vi "Read Roles.vi"(8 "error in (no error)":errorcluster, 11 "KickPenaltyAllyPlay in":refnum<class "KickPenaltyAllyPlay.lvclass">) -> (0 "error out":errorcluster, 2 "Roles":T1, 3 "KickPenaltyAllyPlay out":refnum<class "KickPenaltyAllyPlay.lvclass">)   [LabVIEW 2023, in "KickPenaltyAllyPlay.lvclass"]
uses:
  KickPenaltyAllyPlay.lvclass
  kickPenaltyAllyRoles.ctl
  PenaltyAttackerRole_class/PenaltyAttackerRole.lvclass
  HaltRole_class/HaltRole.lvclass
  KickPenaltyAllyPlay.lvclass/KickPenaltyAllyPlay.ctl
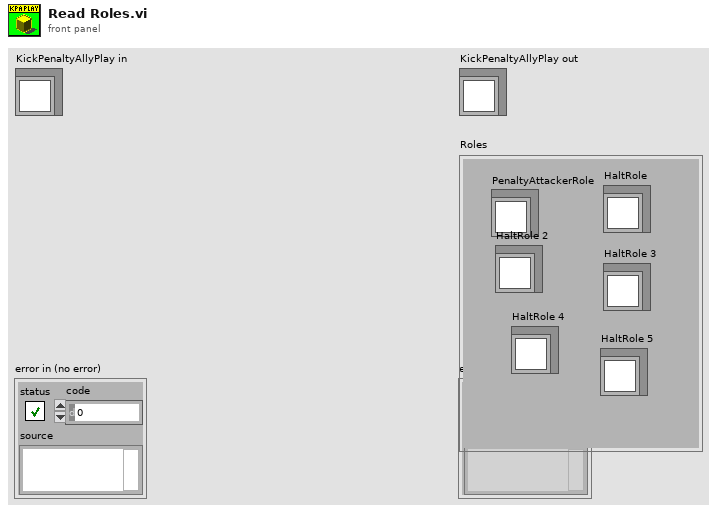
[diagram p1: front panel]
types:
  T1 = typedef "kickPenaltyAllyRoles.ctl" = cluster{"PenaltyAttackerRole":refnum<class "PenaltyAttackerRole.lvclass">, "HaltRole":refnum<class "HaltRole.lvclass">, "HaltRole 2":refnum<class "HaltRole.lvclass">, "HaltRole 3":refnum<class "HaltRole.lvclass">, "HaltRole 4":refnum<class "HaltRole.lvclass">, "HaltRole 5":refnum<class "HaltRole.lvclass">}
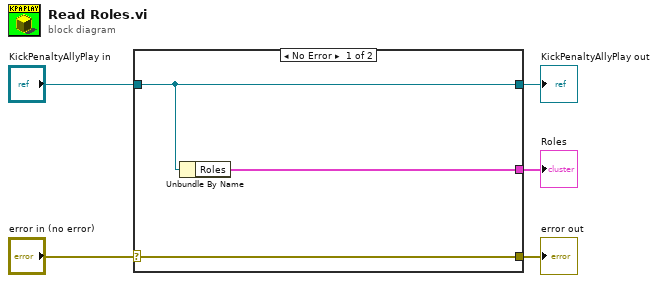
[diagram p0: block diagram]
diagram:
  n1 = case shown="No Error" "error in (no error)" {
    selector: "error in (no error)" -> [w8 w9]
    tunnel: [w8 w9] -> w4
    tunnel: [w7 w10] -> w2
    tunnel: "KickPenaltyAllyPlay in" -> [w7 w10]
    tunnel: [w6 _] -> w1
    frame No Error {
      n2 = Unbundle By Name(w7) -> ("Roles"=w6:T1)
    }
    frame Error {
    }
  }
  "error out" <- w4
  "KickPenaltyAllyPlay out" <- w2
  "Roles" <- w1
